vi "Write Mode.vi"(8 "error in":errorcluster, 10 "Mode":T1, 11 "Electronic Load in":refnum<class "Electronic Load.lvclass">) -> (0 "error out":errorcluster, 3 "Electronic Load out":refnum<class "Electronic Load.lvclass">)   [LabVIEW 2019, in "Electronic Load.lvlib" / "Electronic Load.lvclass"]
uses:
  Library/Electronic Load.lvclass
  C:/Users/Public/Documents/Development/builds/Instruments/Instruments.lvlibp/Library/Instruments.lvclass
  Custom Controls/E-Load Mode.ctl
  Library/Electronic Load.lvclass/Electronic Load.ctl
  builds/Instruments/Instruments.lvlibp/Private/Polymorphic/Special/Event from Enum.vi
  builds/Instruments/Instruments.lvlibp/Accessors/Command with Logging.vi
  builds/Instruments/Instruments.lvlibp/Library/Instruments.lvclass
  builds/Instruments/Instruments.lvlibp
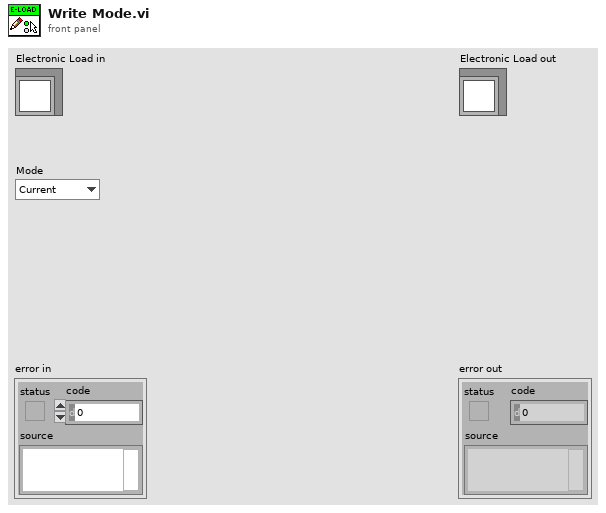
[diagram p1: front panel]
types:
  T1 = typedef "Electronic Load.lvlib/Electronic Load.lvclass/E-Load Mode.ctl" = enum16{"Current", "Resistance", "Voltage"}
  T2 = typedef "Electronic Load.lvlib/Electronic Load.lvclass/E-Load Function.ctl" = cluster{"Mode":T1, "Input Level":dbl, "Output":bool, "Slew Rate":dbl}
  T3 = cluster{"Timestamp":timestamp, "Description":string, "Data":string}
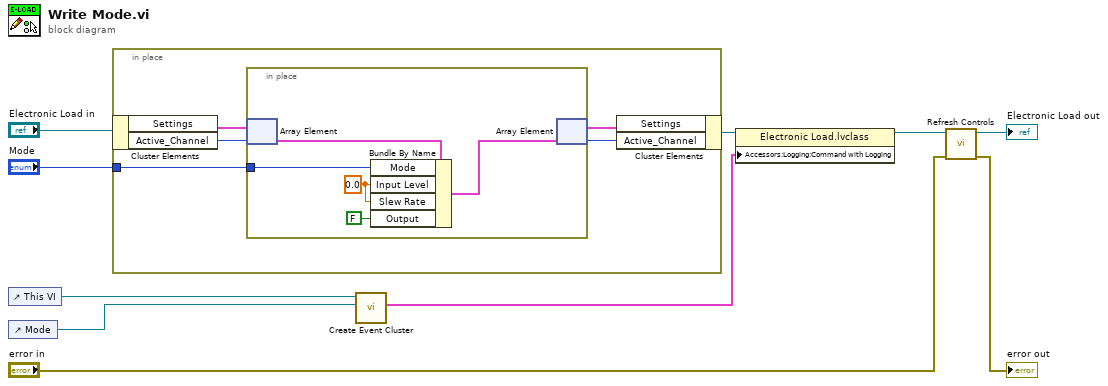
[diagram p0: block diagram]
diagram:
  n1 = control-ref of="This VI"() -> (w7:refnum<vi>)
  n2 = control-ref of="Mode"() -> (w6:refnum<vi>)
  n3 = in-place {
    in-place-border: "Mode" -> [w11]
    n4 = in-place-cluster #1("Electronic Load in") -> ("Settings"=w15:T2[], "Active_Channel"=w14:u32)
    n5 = in-place {
      in-place-border: w11 -> [w18]
      w17 = 0.0 ("Input Level")
      n6 = in-place-array #2(w15, w14) -> (w20:T2)
      n7 = Bundle By Name(cluster=w20, "Mode"=w18, "Input Level"=w17, "Slew Rate"=w17, "Output"=FALSE) -> (w19:T2)
      n8 = in-place-array #2(w19) -> (w13:T2[], w12:i32)
    }
    n9 = in-place-cluster #1("Settings"=w13, "Active_Channel"=w12) -> (w8:refnum<class "Electronic Load.lvclass">)
  }
  n10 = call-poly "Create Event Cluster.vi"("Value"=w6, "VI Refnum"=w7) -> ("Event Data"=w5:T3)  [unwired: 9 in]
  n11 = property class="Electronic Load.lvclass"(reference=w8, "Accessors:Logging:Command with Logging"=w5) -> (reference out=w4:refnum<class "Electronic Load.lvclass">)  [unwired: 1 in, 1 out]
  n12 = call "Refresh Controls.vi"("error in"="error in", "Electronic Load in"=w4) -> ("error out"=→"error out":errorcluster, "Electronic Load out"=→"Electronic Load out":refnum<class "Electronic Load.lvclass">)  [unwired: 8 in]
